vi "Unregister and Destroy Sessions.vi"(8 "error in (no error)":errorcluster) -> (0 "error out":errorcluster)   [LabVIEW 2020, in "Keysight 34401A DMM Measurement.lvlib"]
uses:
  Keysight 34401A DMM Measurement.lvlib
  <vilib>/MeasurementLink/MeasurementLink Discovery Client/RPC Messages/ni_measurementlink_discovery_v1_ResolveServiceRequest.ctl
  <vilib>/MeasurementLink/MeasurementLink Session Management Client/RPC Messages/ni_measurementlink_sessionmanagement_v1_ReserveAllRegisteredSessionsRequest.ctl
  <vilib>/MeasurementLink/MeasurementLink Session Management Client/MeasurementLink Session Management Client.lvlib
  <vilib>/MeasurementLink/MeasurementLink Discovery Client/MeasurementLink Discovery Client.lvlib
  <vilib>/MeasurementLink/MeasurementLink Measurement Server/MeasurementLink Measurement Server.lvlib
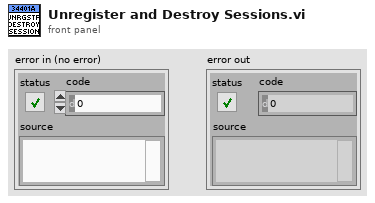
[diagram p1: front panel]
types:
  T1 = typedef "MeasurementLink Session Management Client.lvlib/ni_measurementlink_sessionmanagement_v1_ReserveAllRegisteredSessionsRequest.ctl" = cluster{"timeout_in_milliseconds":i32, "instrument_type_id":string}
  T2 = typedef "MeasurementLink Discovery Client.lvlib/ni_measurementlink_discovery_v1_ResolveServiceRequest.ctl" = cluster{"provided_interface":string, "service_class":string}
  T3 = typedef "grpc-lvsupport-release.lvlib/grpcId.ctl" = u64
  T4 = typedef "MeasurementLink Discovery Client.lvlib/ni_measurementlink_discovery_v1_ServiceLocation.ctl" = cluster{"location":string, "insecure_port":string, "ssl_authenticated_port":string}
  T5 = typedef "MeasurementLink Session Management Client.lvlib/ni_measurementlink_sessionmanagement_v1_ReserveAllRegisteredSessionsResponse.ctl" = cluster{"sessions":T6[]}
  T6 = typedef "MeasurementLink Session Management Client.lvlib/ni_measurementlink_sessionmanagement_v1_SessionInformation.ctl" = cluster{"session":T7, "resource_name":string, "channel_list":string, "instrument_type_id":string, "session_exists":bool, "channel_mappings":T8[]}
  T7 = typedef "MeasurementLink Session Management Client.lvlib/nidevice_grpc_Session.ctl" = cluster{"name":string}
  T8 = typedef "MeasurementLink Session Management Client.lvlib/ni_measurementlink_sessionmanagement_v1_ChannelMapping.ctl" = cluster{"pin_or_relay_name":string, "site":i32, "channel":string}
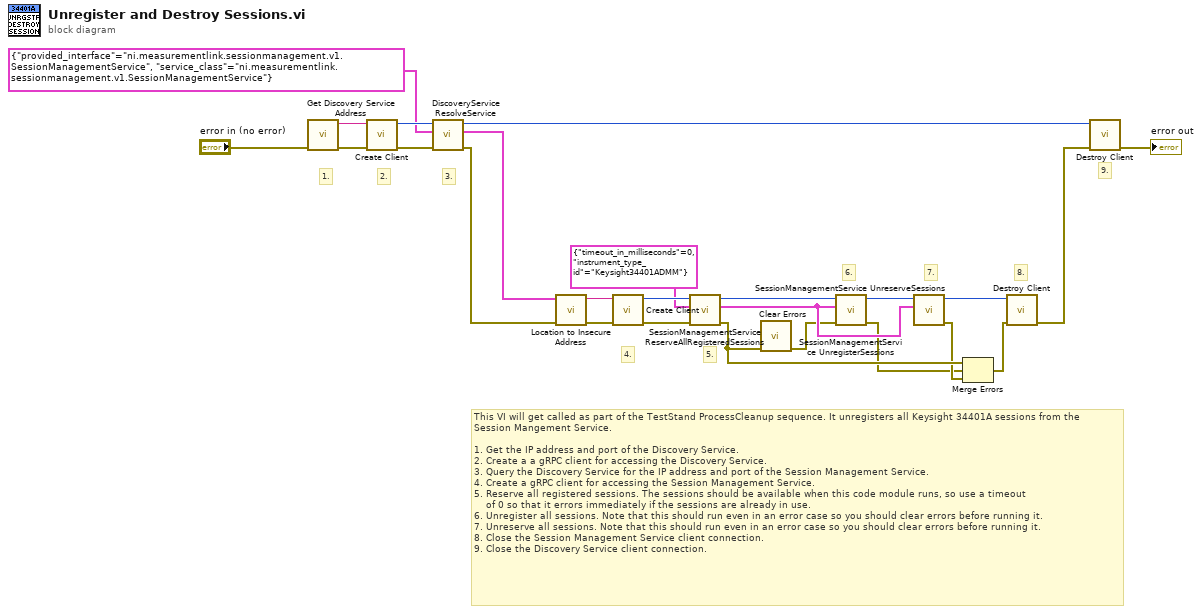
[diagram p0: block diagram]
diagram:
  # "9."
  # "8."
  # "7."
  # "6."
  # "5."
  # "4."
  # "3."
  # "2."
  # "1."
  # "This VI will get called as part of the TestStand ProcessCleanup sequence. It unregisters all Keysight 34401A sessions from the\nSession Mangement Service.\n\n1. Get the IP address and port of the Discovery Service.\n2. Create a a gRPC client for accessing the Discovery Service.\n3. Query the Discovery Service for the IP address and port of the Session Management Service.\n4. Create a gRPC client for accessing the Session Management Service.\n5. Reserve all registered sessions. The sessions should be available when this code module runs, so use a timeout\n    of 0 so that it errors immediately if the sessions are already in use. \n6. Unregister all sessions. Note that this should run even in an error case so you should clear errors before running it.\n7. Unreserve all sessions. Note that this should run even in an error case so you should clear errors before running it.\n8. Close the Session Management Service client connection.\n9. Close the Discovery Service client connection."
  n1 = call <vilib>:"Get Discovery Service Address.vi"("error in"="error in (no error)") -> ("error out"=w11:errorcluster, "address"=w10:string)  [unwired: 9 in]
  n2 = call <vilib>:"Create Client.vi"("error in"=w11, "address"=w10) -> ("error out"=w23:errorcluster, "gRPC ID Out"=w24:T3)  [unwired: 8 in]
  n3 = call <vilib>:"DiscoveryService ResolveService.vi"("error in"=w23, "Request Data"=T2 {"provided_interface"="ni.measurementlink.sessionmanagement.v1.SessionManagementService", "service_class"="ni.measurementlink.sessionmanagement.v1.SessionManagementService"}, "gRPC ID"=w24) -> ("error out"=w8:errorcluster, "Response Data"=w7:T4, "gRPC ID out"=w18:T3)  [unwired: 6 in]
  n4 = call "Location to Insecure Address.vi"("Response Data"=w7) -> ("String"=w6:string)  [unwired: 10 in]
  n5 = call <vilib>:"Create Client.vi"("error in"=w8, "address"=w6) -> ("error out"=w17:errorcluster, "gRPC ID Out"=w16:T3)  [unwired: 8 in]
  n6 = call <vilib>:"SessionManagementService ReserveAllRegisteredSessions.vi"("error in"=w17, "Request Data"=T1 {"timeout_in_milliseconds"=0, "instrument_type_id"="Keysight34401ADMM"}, "gRPC ID"=w16) -> ("error out"=w14:errorcluster, "Response Data"=w5:T5, "gRPC ID out"=w13:T3)  [unwired: 6 in]
  n7 = call <vilib>:"Clear Errors.vi"("error in (no error)"=w14) -> ("error out"=w1:errorcluster)  [unwired: 5 in, 1 out]
  n8 = call <vilib>:"SessionManagementService UnregisterSessions.vi"("error in"=w1, "Request Data"=w5, "gRPC ID"=w13) -> ("error out"=w2:errorcluster, "gRPC ID out"=w12:T3)  [unwired: 6 in, 1 out]
  n9 = call <vilib>:"SessionManagementService UnreserveSessions.vi"("Request Data"=w5, "gRPC ID"=w12) -> ("error out"=w4:errorcluster, "gRPC ID out"=w19:T3)  [unwired: 7 in, 1 out]
  n10 = Merge Errors(w14, w2, w4) -> (w3:errorcluster)
  n11 = call <vilib>:"Destroy Client.vi"("error in"=w3, "gRPC ID"=w19) -> ("error out"=w22:errorcluster)  [unwired: 9 in]
  n12 = call <vilib>:"Destroy Client.vi"("error in"=w22, "gRPC ID"=w18) -> ("error out"=→"error out":errorcluster)  [unwired: 9 in]
